vi "Read Elevator Call.vi"(8 "error in (no error)":errorcluster, 11 "Sim User Console Actor in":refnum<class "Sim User Console Actor.lvclass">) -> (0 "error out":errorcluster, 3 "Sim User Console Actor out":refnum<class "Sim User Console Actor.lvclass">)   [LabVIEW 2022 SP3, in "Sim User Console Actor.lvlib" / "Sim User Console Actor.lvclass"]
uses:
  Sim User Console Actor.lvclass
  Sim User Console Actor.lvclass/Sim User Console Actor.ctl
  Interface Elevator/Interface Elevator Msg/Set State Msg/Set State Msg.lvclass
  <vilib>/ActorFramework/Actor/Actor.lvclass
  Elevator Controller Actor/Elevator Controller Actor/State -Enum.ctl
  Elevator Controller Actor/Elevator Controller Actor/Elevator Controller Actor.lvclass
  C:/Workspace/CLA/Elevator AF_2022_2nd/User Console Actor/User Console Actor/User Console Actor.lvclass
  C:/Program Files/National Instruments/LabVIEW 2022/vi.lib/ActorFramework/Actor/Actor.lvclass
  C:/Workspace/CLA/Elevator AF_2022_2nd/Sim User Console Actor/Elevator Controller Actor/Sim User Console Actor.lvclass
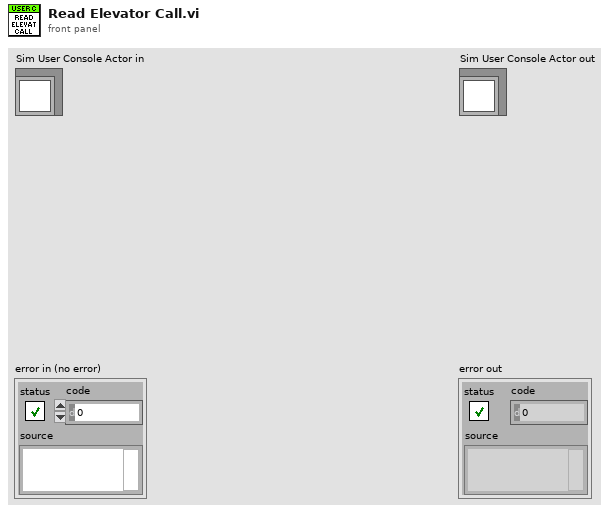
[diagram p1: front panel]
types:
  T1 = typedef "Elevator Controller Actor.lvlib/Elevator Controller Actor.lvclass/State -Enum.ctl" = enum16{"Initial", "Wait for First Request", "Start and Move", "Anaysis", "Continue Travel", "Stop at Floor", "Open and Close Door Sequence", "No Request Remaining", "Emergency Call", "Terminate Process"}
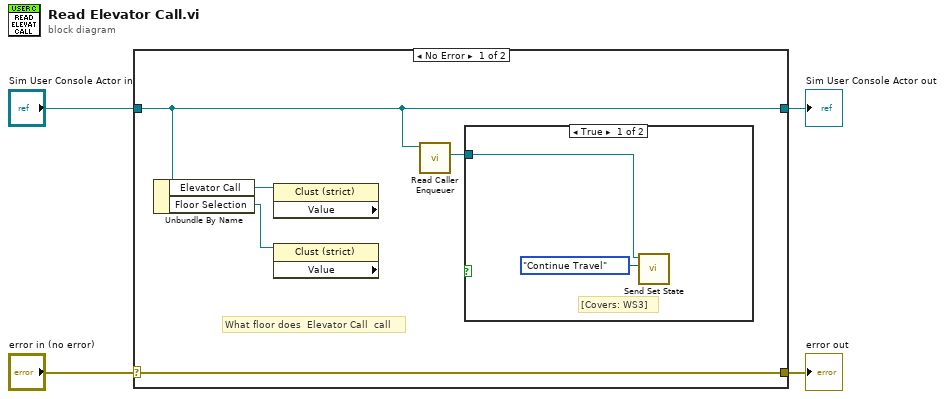
[diagram p0: block diagram]
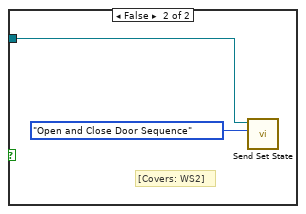
[diagram p2: hidden frame]
diagram:
  n1 = case shown="No Error" "error in (no error)" {
    selector: "error in (no error)" -> [w9 w15]
    tunnel: [w9 w15] -> w3
    tunnel: [w6 w14] -> w1
    tunnel: "Sim User Console Actor in" -> [w6 w14]
    frame No Error {
      # "What floor does  Elevator Call  call"
      n2 = Unbundle By Name(w6) -> ("Elevator Call"=w8:refnum<vi>, "Floor Selection"=w7:refnum<vi>)
      n3 = property class="Clust (strict)" props=["Value"](reference=w8) -> ()  [unwired: 1 in, 3 out]
      n4 = property class="Clust (strict)" props=["Value"](reference=w7) -> ()  [unwired: 1 in, 3 out]
      n5 = call <vilib>:"Read Caller Enqueuer.vi"("Actor"=w6) -> ("Caller Enqueuer"=w5:refnum<class "Message Enqueuer.lvclass">)  [unwired: 10 in]
      n6 = case shown="\"another floor\"" {
        selector: _ -> [_ _]
        tunnel: w5 -> [w11 w13]
        frame True {
          # "[Covers: WS3]"
          n7 = call "Send Set State.vi"("State"=State_-Enum."Continue Travel", "Message Enqueuer"=w11) -> ()  [unwired: 8 in, 2 out]
        }
        frame False {
          # "[Covers: WS2]"
          n8 = call "Send Set State.vi"("State"=State_-Enum."Open and Close Door Sequence", "Message Enqueuer"=w13) -> ()  [unwired: 8 in, 2 out]
        }
      }
    }
    frame Error {
    }
  }
  "error out" <- w3
  "Sim User Console Actor out" <- w1
